vi "Number Of LBCBs 2 Sources.vi"(2 "Number of LBCBs":T2, 3 "Combined LBCBs":bool) -> (0 "Source Text":string[](array[string]), 1 "Sources":T1[](array[typedef]))   [LabVIEW 2013]
uses:
  Data Access Objects/Application/Number Of LBCBs.ctl
  W:/NSEL OM/lib/Global Data/Names/Source Group Type.ctl
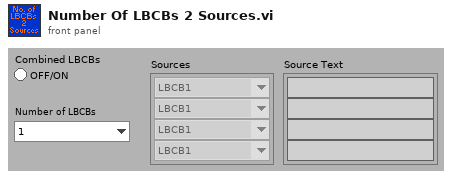
[diagram p1: front panel]
types:
  T1 = typedef "Source Group Type.ctl" = enum16{"LBCB1", "LBCB2", "Consolidated", "External"}
  T2 = typedef "Number Of LBCBs.ctl" = enum16{"1", "2"}
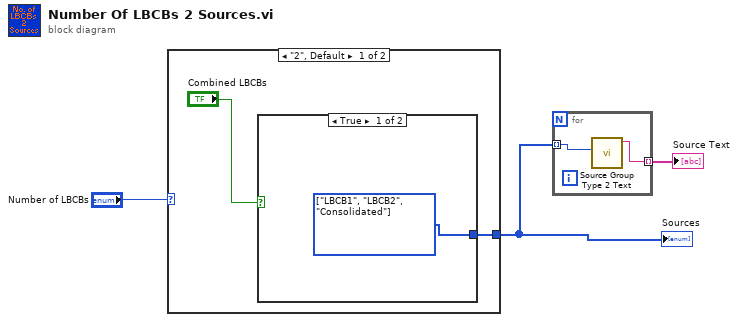
[diagram p0: block diagram]
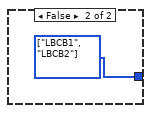
[diagram p2: hidden frame]
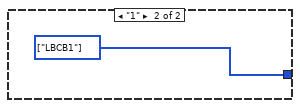
[diagram p3: hidden frame]
diagram:
  n1 = case shown="\"2\", Default" "Number of LBCBs" {
    tunnel: [w5 w8] -> w2
    frame "2", Default {
      n2 = case shown="True" "Combined LBCBs" {
        tunnel: [w6 w7] -> w5
        frame True {
          w6 = T1[] [enum."LBCB1", enum."LBCB2", enum."Consolidated"] items=["LBCB1", "LBCB2", "Consolidated", "External"]
        }
        frame False {
          w7 = T1[] [enum."LBCB1", enum."LBCB2"] items=["LBCB1", "LBCB2", "Consolidated", "External"]
        }
      }
    }
    frame "1" {
      w8 = T1[] [enum."LBCB1"] items=["LBCB1", "LBCB2", "Consolidated", "External"]
    }
  }
  "Sources" <- w2
  n3 = for {
    tunnel: w2 -> [w10] mode=indexing
    tunnel: [w9] -> w1 mode=indexing
    n4 = call "Source Group Type 2 Text.vi"("Source"=w10) -> ("String"=w9:string)  [unwired: 10 in]
  }
  "Source Text" <- w1
